vi "Read path.vi"(8 "error in (no error)":errorcluster, 11 "Generic Client in":refnum<class "Generic Client.lvclass">) -> (0 "error out":errorcluster, 2 "path":path, 3 "Generic Client out":refnum<class "Generic Client.lvclass">)   [LabVIEW 2020, in "NI_SSH.lvlib" / "Generic Client.lvclass"]
uses:
  <vilib>/net/SSH/Client/Generic/Generic Client.lvclass
  <vilib>/net/SSH/Client/Generic/Generic Client.lvclass/Generic Client.ctl
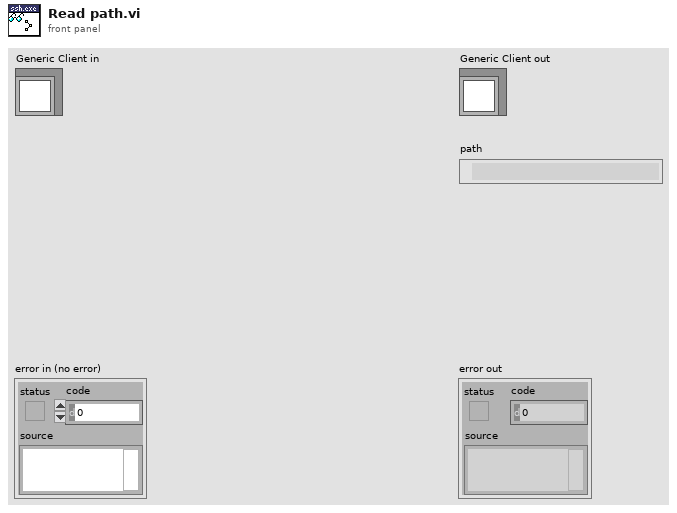
[diagram p1: front panel]
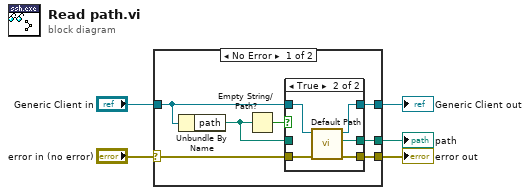
[diagram p0: block diagram]
diagram:
  n1 = case shown="No Error" "error in (no error)" {
    selector: "error in (no error)" -> [w8 w21]
    tunnel: [w7 w21] -> w4
    tunnel: [w10 w22] -> w2
    tunnel: "Generic Client in" -> [w9 w22]
    tunnel: [w6 _] -> w1
    frame No Error {
      n2 = Unbundle By Name(w9) -> ("path"=w11:path)
      n3 = Empty String/Path?(string/path=w11) -> (empty?=w12:bool)
      n4 = case shown="True" w12 {
        tunnel: w9 -> [w13 w20]
        tunnel: [w15 w17] -> w6
        tunnel: w11 -> [w15 _]
        tunnel: w8 -> [w14 w19]
        tunnel: [w14 w16] -> w7
        tunnel: [w13 w18] -> w10
        frame False {
        }
        frame True {
          n5 = call-dynamic "Default Path.vi"("error in (no error)"=w19, "Generic Client in"=w20) -> ("error out"=w16:errorcluster, "path"=w17:path, "Generic Client out"=w18:refnum<class "Generic Client.lvclass">)  [unwired: 7 in]
        }
      }
    }
    frame Error {
    }
  }
  "error out" <- w4
  "Generic Client out" <- w2
  "path" <- w1
